vi "open_curves.vi"(2 "error in (no error)":errorcluster, 3 "Path":path) -> (0 "error out":errorcluster, 1 "All TXT files":path[](array[path]))   [LabVIEW 2015]
panel:
  out "All Files in Dir":path[](array[path])
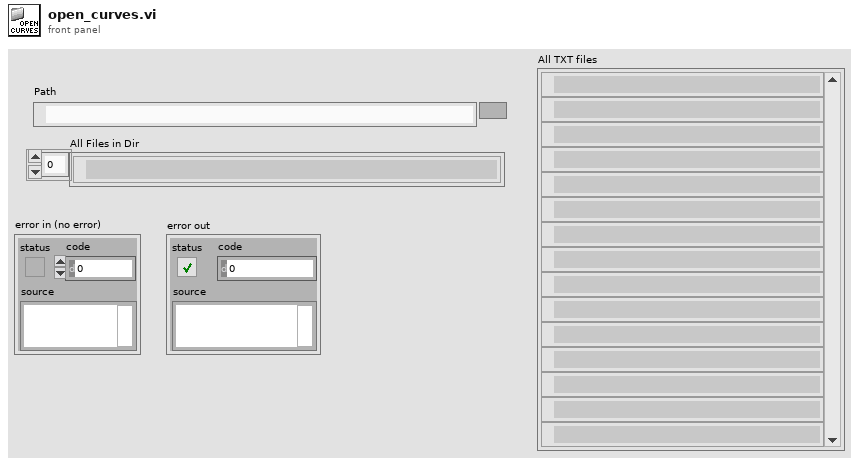
[diagram p1: front panel]
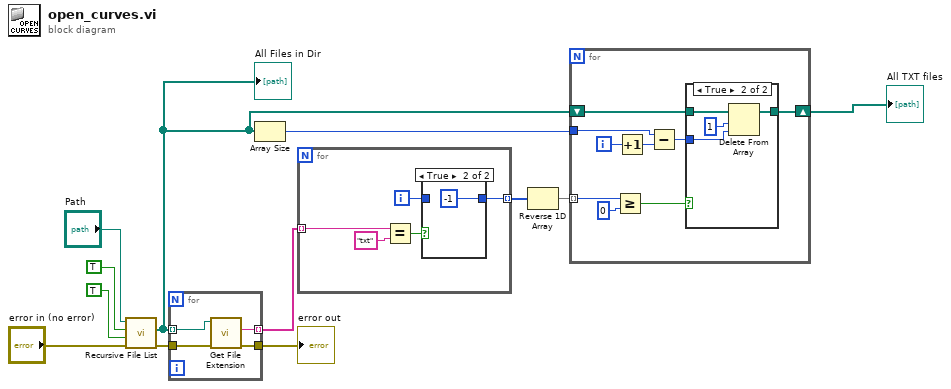
[diagram p0: block diagram]
diagram:
  n1 = call <vilib>:"Recursive File List.vi"("error in (no error)"="error in (no error)", "Continue Recursing on Error? (F)"=TRUE, "Treat LLBs as Folders?"=TRUE, "Folder Path"="Path") -> ("error out"=w2:errorcluster, "All Files in Dir"=w6:path[])  [unwired: 3 in, 3 out]
  "All Files in Dir" <- w6
  n2 = for {
    tunnel: w6 -> [w16] mode=indexing
    tunnel: [w15] -> w9 mode=indexing
    tunnel: w2 -> [w14]
    tunnel: [w13] -> w1
    n3 = call <vilib>:"Get File Extension.vi"("error in (no error)"=w14, "file"=w16) -> ("error out"=w13:errorcluster, "lowercase file extension"=w15:string)  [unwired: 5 in, 3 out]
  }
  "error out" <- w1
  n4 = Array Size(array=w6) -> (size(s)=w5:i32)
  n5 = for {
    tunnel: w9 -> [w21] mode=indexing
    tunnel: [w18] -> w8 mode=indexing
    i -> [w17]
    n6 = Equal?(x=w21, y="txt") -> (x = y?=w19:bool)
    n7 = case shown="True" w19 {
      tunnel: w17 -> [w22 _]
      tunnel: [w22 -1] -> w18
      frame False {
      }
      frame True {
      }
    }
  }
  n8 = Reverse 1D Array(array=w8) -> (reversed array=w7:i32[])
  n9 = for {
    shift-right: [w29] -> w4
    shift-left: w6 -> [w30]
    tunnel: w7 -> [w28] mode=indexing
    tunnel: w5 -> [w27]
    i -> [w25]
    n10 = Greater Or Equal?(x=w28, y=0) -> (x >= y?=w31:bool)
    n11 = Increment(x=w25) -> (x+1=w24:i32)
    n12 = Subtract(x=w27, y=w24) -> (x-y=w26:i32)
    n13 = case shown="True" w31 {
      tunnel: w30 -> [w33 w37]
      tunnel: [w33 w36] -> w29
      tunnel: w26 -> [_ w35]
      frame False {
      }
      frame True {
        n14 = Delete From Array(array=w37, length=1, index=w35) -> (array with subset deleted=w36:path[])  [unwired: 1 out]
      }
    }
  }
  "All TXT files" <- w4
